vi "Interface_Asset_Process.vi"(8 "error in (no error)":errorcluster, 10 "data value reference":refnum<data-value>, 11 "Grid in":refnum<class "Grid.lvclass">) -> ()   [LabVIEW 2015, in "Grid.lvclass"]
uses:
  Grid.lvclass
  Interface_Asset/Interface_Asset.lvclass
  Grid.lvclass/Grid.ctl
panel:
  in  "stop":bool
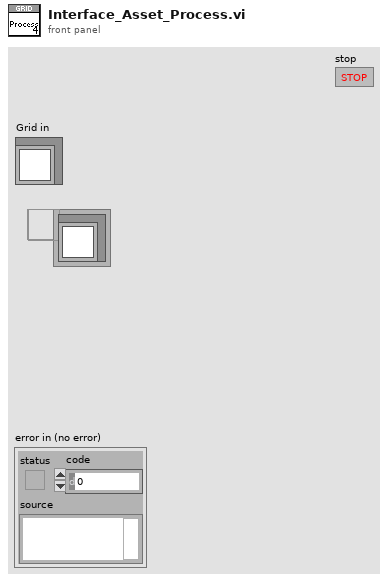
[diagram p1: front panel]
types:
  T1 = typedef "Grid.lvclass/Grid_Status.ctl" = cluster{"kW":dbl}
  T2 = typedef "Grid.lvclass/Grid_Control.ctl" = cluster{"Placeholder":dbl}
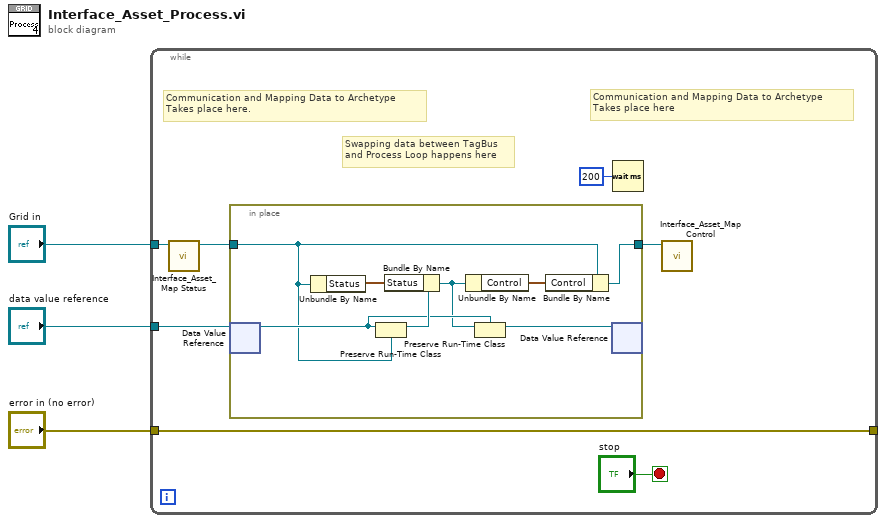
[diagram p0: block diagram]
diagram:
  n1 = while {
    tunnel: "Grid in" -> [w6]
    tunnel: "error in (no error)" -> [w10]
    tunnel: [w10] -> _
    tunnel: "data value reference" -> [w8]
    stop <- "stop" stop-if-true
    # "Swapping data between TagBus\nand Process Loop happens here"
    # "Communication and Mapping Data to Archetype\nTakes place here"
    # "Communication and Mapping Data to Archetype\nTakes place here."
    n2 = call-dynamic "Interface_Asset_Map Status.vi"("Grid in"=w6) -> ("Grid out"=w5:refnum<class "Grid.lvclass">)  [unwired: 9 in, 1 out]
    n3 = in-place {
      in-place-border: w5 -> [w11]
      in-place-border: [w13] -> w4
      n4 = in-place-dvr #1(w8) -> (w15:refnum<class "Interface_Asset.lvclass">)  [unwired: 1 out]
      n5 = Unbundle By Name(w11) -> ("Status"=w18:T1)
      n6 = Preserve Run-Time Class(object in=w15, 2:w11) -> (object out=w17:refnum<class "Grid.lvclass">)  [unwired: 1 in, 1 out]
      n7 = Bundle By Name(cluster=w17, "Status"=w18) -> (w14:refnum<class "Grid.lvclass">)
      n8 = Unbundle By Name(w14) -> ("Control"=w12:T2)
      n9 = Preserve Run-Time Class(object in=w14, 2:w15) -> (object out=w16:refnum<class "Interface_Asset.lvclass">)  [unwired: 1 in, 1 out]
      n10 = Bundle By Name(cluster=w11, "Control"=w12) -> (w13:refnum<class "Grid.lvclass">)
      n11 = in-place-dvr #1(w16) -> ()  [unwired: 2 out]
    }
    n12 = Wait (ms)(milliseconds to wait=u32 200) -> ()  [unwired: 1 out]
    n13 = call-dynamic "Interface_Asset_Map Control.vi"("Grid in"=w4) -> ()  [unwired: 9 in, 2 out]
  }
